vi "ErrorIfNotInitialized.vi"(8 "error in (no error)":errorcluster, 11 "IAmGLF in":refnum<class "IAmGLF.lvclass">) -> (0 "error out":errorcluster, 3 "IAmGLF out":refnum<class "IAmGLF.lvclass">)   [LabVIEW 2020, in "GLF.lvlib" / "IAmGLF.lvclass"]
uses:
  IAmGLF.lvclass
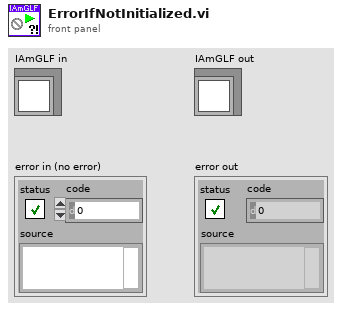
[diagram p1: front panel]
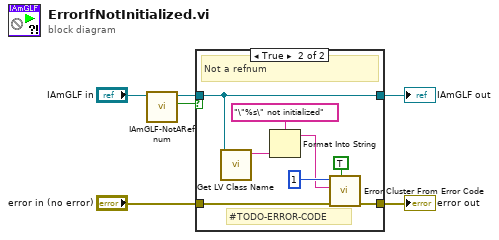
[diagram p0: block diagram]
diagram:
  n1 = call-dynamic "IAmGLF-NotARefnum.vi"("IAmGLF in"="IAmGLF in") -> ("Not A Valid Refnum?"=w6:bool, "IAmGLF out"=w1:refnum<class "IAmGLF.lvclass">)  [unwired: 9 in]
  n2 = case shown="True" w6 {
    tunnel: "error in (no error)" -> [w8 w12]
    tunnel: [w8 w16] -> w3
    tunnel: [w7 w13] -> w2
    tunnel: w1 -> [w7 w13]
    frame False {
      # "Is a Refnum"
    }
    frame True {
      # "#TODO-ERROR-CODE"
      # "Not a refnum"
      n3 = call <vilib>:"Get LV Class Name.vi"("object"=w13) -> ("class name"=w10:string)  [unwired: 9 in, 1 out]
      n4 = Format Into String(format string="\"%s\" not initialized" ("error message (\"\")"), w10) -> (resulting string=w11:string)  [unwired: 2 in, 1 out]
      n5 = call <vilib>:"Error Cluster From Error Code.vi"("show call chain? (False)"=TRUE, "error in (no error)"=w12, "error message (\"\")"=w11, "error code (0)"=1) -> ("error out"=w16:errorcluster)  [unwired: 5 in]
    }
  }
  "error out" <- w3
  "IAmGLF out" <- w2
